vi "Channel Names.vi"(8 "error in (no error)":errorcluster, 11 "DataHandlerTask in":refnum<class "DataHandlerTask.lvclass">) -> (0 "error out":errorcluster, 2 "Channel Names":string[](array[string]), 3 "DataHandlerTask out":refnum<class "DataHandlerTask.lvclass">)   [LabVIEW 2020, in "VolatusData.lvlib" / "DataHandlerTask.lvclass"]
uses:
  DataHandlerTask.lvclass
  DataHandlerTask.lvclass/DataHandlerTask.ctl
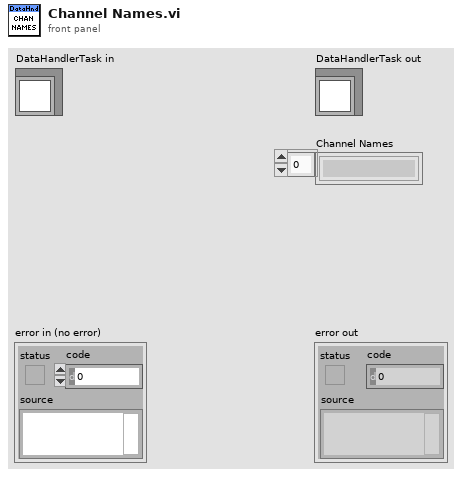
[diagram p1: front panel]
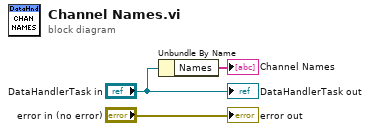
[diagram p0: block diagram]
diagram:
  n1 = Unbundle By Name("DataHandlerTask in") -> ("Names"=→"Channel Names":string[])
  "error out" <- "error in (no error)"
  "DataHandlerTask out" <- "DataHandlerTask in"
